vi "Process.vi"(8 "error in":errorcluster, 11 "server in":refnum<class "RT FlexRIO Server TCP.lvclass">) -> (0 "error out":errorcluster, 3 "server out":refnum<class "RT FlexRIO Server TCP.lvclass">)   [LabVIEW 2017, in "RT FlexRIO Server TCP.lvclass"]
uses:
  RT FlexRIO Server TCP.lvclass
  Public/State.ctl
  Properties/ProcessStopped_GET.vi
  Properties/State_GET.vi
  Properties/State_SET.vi
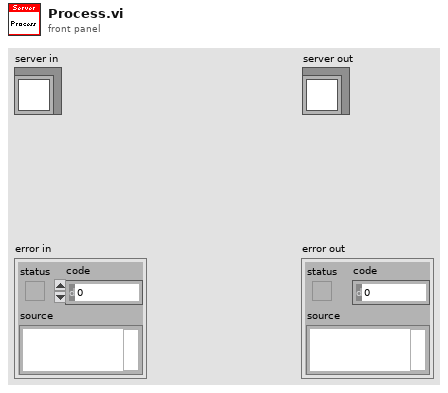
[diagram p1: front panel]
types:
  T1 = typedef "RT FlexRIO Server TCP.lvclass/State.ctl" = enum16{"started", "connected", "stopped"}
  T2 = typedef "RT FlexRIO Server.lvclass/connection state.ctl" = enum16{"started", "connected", "stopped"}
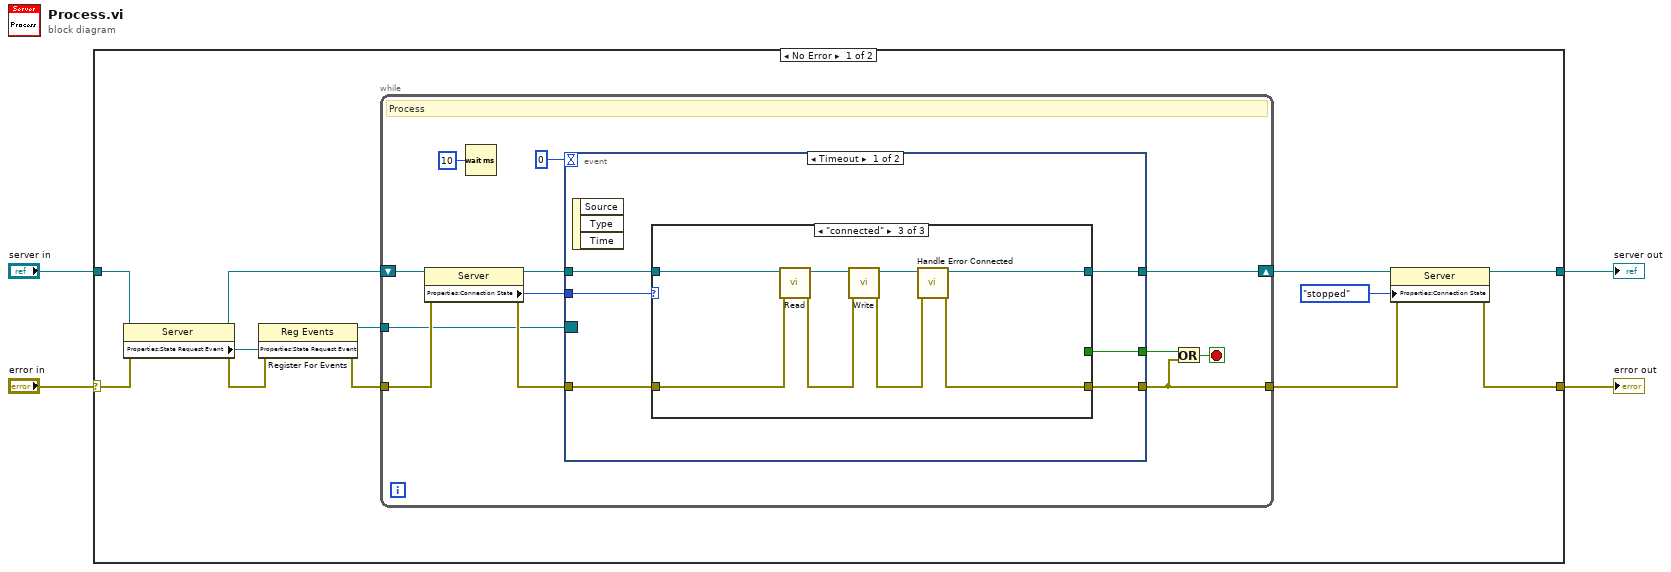
[diagram p0: block diagram]
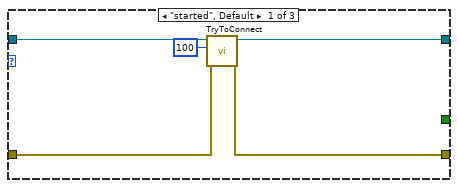
[diagram p2: hidden frame]
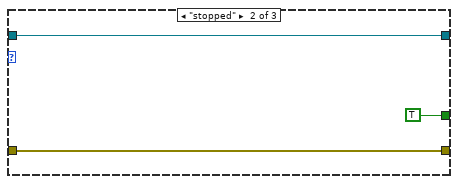
[diagram p3: hidden frame]
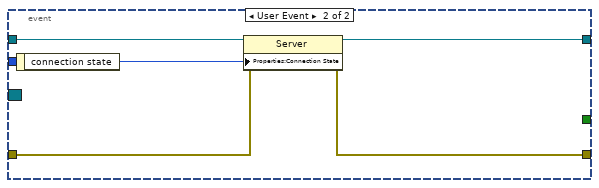
[diagram p4: hidden frame]
diagram:
  n1 = case shown="No Error" "error in" {
    selector: "error in" -> [w13 w56]
    tunnel: "server in" -> [w14 w57]
    tunnel: [w6 w57] -> w2
    tunnel: [w5 w56] -> w1
    frame No Error {
      n2 = property class="Server"(reference=w14, error in=w13) -> (reference out=w7:refnum<class "RT FlexRIO Server TCP.lvclass">, error out=w9:errorcluster, "Properties:State Request Event"=w11:refnum<user-event>)
      n3 = register-events(error in=w9, w11) -> (reference out=w10:refnum<event-registration>, error out=w8:errorcluster)  [unwired: 1 in]
      n4 = while {
        shift-right: [w26] -> w16
        shift-left: w7 -> [w28]
        tunnel: w8 -> [w27]
        tunnel: [w25] -> w12
        tunnel: w10 -> [w20]
        stop <- w24 stop-if-true
        # "Process"
        n5 = property class="Server"(reference=w28, error in=w27) -> (reference out=w21:refnum<class "RT FlexRIO Server TCP.lvclass">, error out=w22:errorcluster, "Properties:Connection State"=w23:T2)
        n6 = Wait (ms)(milliseconds to wait=u32 10) -> ()  [unwired: 1 out]
        n7 = event shown="[0] Timeout" {
          selector: w20 -> [_ _]
          dyn-events: _ -> [_ _]
          timeout: 0 -> [_ _]
          tunnel: [w34 w54] -> w26
          tunnel: [w33 w52] -> w25
          tunnel: w23 -> [w32 _]
          tunnel: w22 -> [w31 w53]
          tunnel: w21 -> [w30 w55]
          tunnel: [w29 _] -> w18
          event Timeout {
            n8 = event-data() -> ()  [unwired: 1 in, 3 out]
            n9 = case shown="\"connected\"" w32 {
              tunnel: w31 -> [w38 w41 w49]
              tunnel: w30 -> [w39 w42 w50]
              tunnel: [w37 w42 w45] -> w34
              tunnel: [w36 w41 w43] -> w33
              tunnel: [_ TRUE _] -> w29
              frame "started", Default {
                n10 = call "TryToConnect.vi"("error in"=w38, "timeout"=100, "server in"=w39) -> ("error out"=w36:errorcluster, "server out"=w37:refnum<class "RT FlexRIO Server TCP.lvclass">)  [unwired: 7 in]
              }
              frame "stopped" {
              }
              frame "connected" {
                n11 = call "Read.vi"("error in"=w49, "tcp server in"=w50) -> ("error out"=w47:errorcluster, "tcp server out"=w48:refnum<class "RT FlexRIO Server TCP.lvclass">)  [unwired: 8 in]
                n12 = call "Write.vi"("error in"=w47, "server in"=w48) -> ("error out"=w44:errorcluster, "server out"=w46:refnum<class "RT FlexRIO Server TCP.lvclass">)  [unwired: 8 in]
                n13 = call "Handle Error Connected.vi"("error in"=w44, "server in"=w46) -> ("error out"=w43:errorcluster, "server out"=w45:refnum<class "RT FlexRIO Server TCP.lvclass">)  [unwired: 8 in]
              }
            }
          }
          event User Event {
            n14 = event-data() -> ("connection state"=w51:T2)  [unwired: 1 in]
            n15 = property class="Server"(reference=w55, error in=w53, "Properties:Connection State"=w51) -> (reference out=w54:refnum<class "RT FlexRIO Server TCP.lvclass">, error out=w52:errorcluster)
          }
        }
        n16 = Or(x=w18, y=w25) -> (x .or. y?=w24:bool)
      }
      n17 = property class="Server"(reference=w16, error in=w12, "Properties:Connection State"=State."stopped" ("Connection State")) -> (reference out=w6:refnum<class "RT FlexRIO Server TCP.lvclass">, error out=w5:errorcluster)
    }
    frame Error {
    }
  }
  "error out" <- w1
  "server out" <- w2
